vi "_SetPowerState.vi"(8 "error in (no error)":errorcluster, 10 "PowerState":enum16{"Off", "Sleep", "On"}(ring)=enum."Sleep", 11 "CellPhone in":refnum<class "CellPhone.lvclass">) -> (0 "error out":errorcluster, 3 "CellPhone out":refnum<class "CellPhone.lvclass">)   [LabVIEW 2009, in "CellPhone.lvclass"]
uses:
  CellPhone.lvclass
  CellPhone.lvclass/CellPhone.ctl
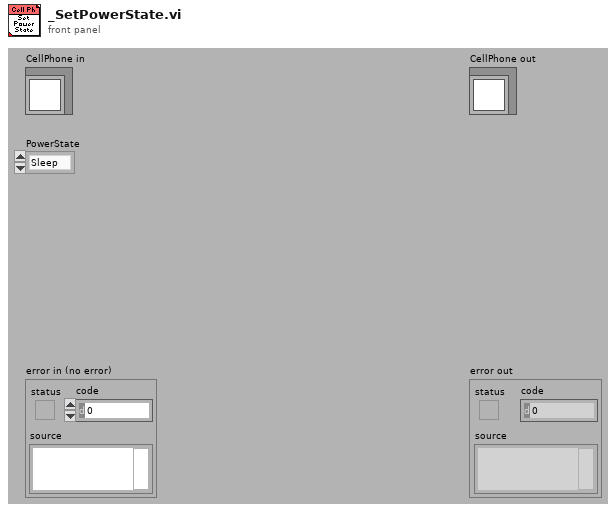
[diagram p1: front panel]
types:
  T1 = typedef "CellPhone.lvclass/_PrivateDataDvr.ctl" = refnum<data-value>
  T2 = typedef "CellPhone.lvclass/_PrivateData.ctl" = cluster{"PowerState":enum16{"Off", "Sleep", "On"}}
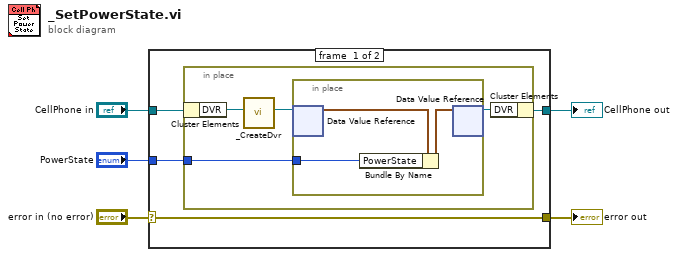
[diagram p0: block diagram]
diagram:
  n1 = case shown="No Error" "error in (no error)" {
    selector: "error in (no error)" -> [w9 w18]
    tunnel: [w9 w18] -> w4
    tunnel: [w7 w17] -> w2
    tunnel: "CellPhone in" -> [w8 w17]
    tunnel: "PowerState" -> [w6 _]
    frame #0 {
      n2 = in-place {
        in-place-border: w6 -> [w10]
        n3 = in-place-cluster #1(w8) -> ("DVR"=w13:T1)
        n4 = call "_CreateDvr.vi"("DVR"=w13) -> ("DVR out"=w12:T1)  [unwired: 10 in]
        n5 = in-place {
          in-place-border: w10 -> [w14]
          n6 = in-place-dvr #2(w12) -> (w16:T2)  [unwired: 1 out]
          n7 = Bundle By Name(cluster=w16, "PowerState"=w14) -> (w15:T2)
          n8 = in-place-dvr #2(w15) -> (w11:T1)  [unwired: 1 out]
        }
        n9 = in-place-cluster #1("DVR"=w11) -> (w7:refnum<class "CellPhone.lvclass">)
      }
    }
    frame #1 {
    }
  }
  "error out" <- w4
  "CellPhone out" <- w2
